vi "IAmGLF-DeleteFromStandaloneProcess.vi"(8 "error in (no error)":errorcluster, 10 "Error Return Notifier":refnum<notifier>, 11 "Engine in":refnum<class "Engine.lvclass">) -> (0 "error out":errorcluster)   [LabVIEW 2024, in "GLF.lvlib" / "Engine.lvclass"]
uses:
  Engine.lvclass
  Engine.lvclass/Engine.ctl
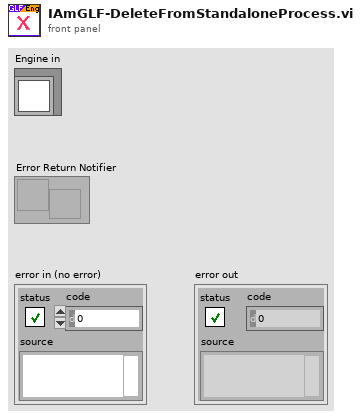
[diagram p1: front panel]
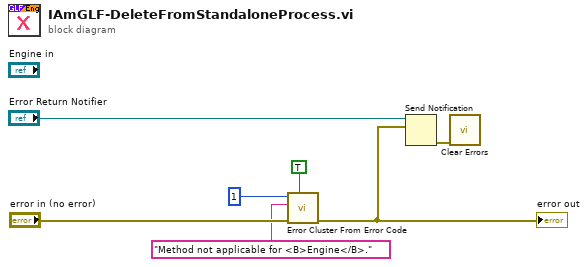
[diagram p0: block diagram]
diagram:
  n1 = call <vilib>:"Error Cluster From Error Code.vi"("show call chain? (False)"=TRUE, "error in (no error)"="error in (no error)", "error message (\"\")"="Method not applicable for <B>Engine</B>." ("error message (\"\")"), "error code (0)"=1) -> ("error out"=w1:errorcluster)  [unwired: 5 in]
  "error out" <- w1
  n2 = Send Notification(notification=w1, notifier="Error Return Notifier") -> (error out=w2:errorcluster)  [unwired: 1 in, 1 out]
  n3 = call <vilib>:"Clear Errors.vi"("error in (no error)"=w2) -> ()  [unwired: 5 in, 2 out]
